vi "WPI_AnalogTriggerVoltsToValue.vi"(8 "error in (no error)":errorcluster, 9 "Voltage":dbl, 10 "AnalogTriggerSource":T1={"Channel"=enum."AI 1", "Averaged"=FALSE, "Filter"=FALSE}, 11 "AnalogTriggerDevRef":T3) -> (0 "error out":errorcluster, 1 "Value":i32, 3 "AnalogTriggerDevRef":T3)   [LabVIEW 2017]
doc: "This software is licensed. Open the labview\\readme\\WPI Robotics Library Open Source License.txt file for more information."
uses:
  <vilib>/Rock Robotics/SystemInterfaces/AnalogTrigger/FPGA_AnalogTriggerDevRef.ctl
  <vilib>/Rock Robotics/SystemInterfaces/AnalogTrigger/FPGA_AnalogTriggerIndex.ctl
  <vilib>/Rock Robotics/SystemInterfaces/AnalogTrigger/FPGA_AnalogTriggerSource.ctl
  <vilib>/Rock Robotics/SystemInterfaces/AI/FPGA_AIChannel.ctl
  <vilib>/Rock Robotics/SystemInterfaces/System/FPGA_SystemGet.vi
  <vilib>/Rock Robotics/SystemInterfaces/AI/FPGA_AIOversampleBits.vi
  <vilib>/Rock Robotics/SystemInterfaces/AI/FPGA_AIERRInvalidAnalogChannel.vi
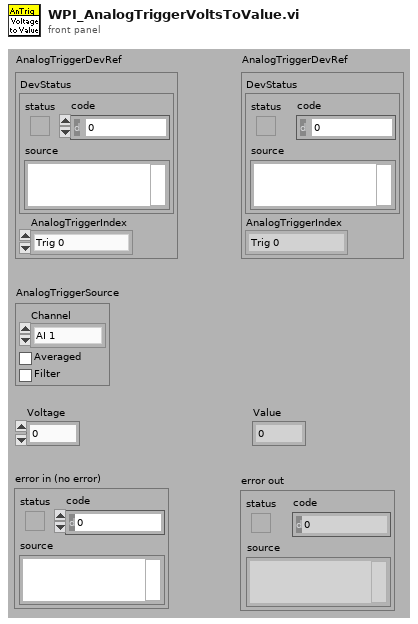
[diagram p1: front panel]
types:
  T1 = typedef "FPGA_AnalogTriggerSource.ctl" = cluster{"Channel":T2, "Averaged":bool, "Filter":bool}
  T2 = typedef "FPGA_AIChannel.ctl" = enum8{"AI 0", "AI 1", "AI 2", "AI 3", "AI MXP 0", "AI MXP 1", "AI MXP 2", "AI MXP 3", "Invalid"}
  T3 = typedef "FPGA_AnalogTriggerDevRef.ctl" = cluster{"DevStatus":errorcluster, "AnalogTriggerIndex":T4}
  T4 = typedef "FPGA_AnalogTriggerIndex.ctl" = enum8{"Trig 0", "Trig 1", "Trig 2", "Trig 3", "Trig 4", "Trig 5", "Trig 6", "Trig 7", "Invalid"}
  T5 = typedef "FPGA_AIDevRef.ctl" = cluster{"DevStatus":errorcluster}
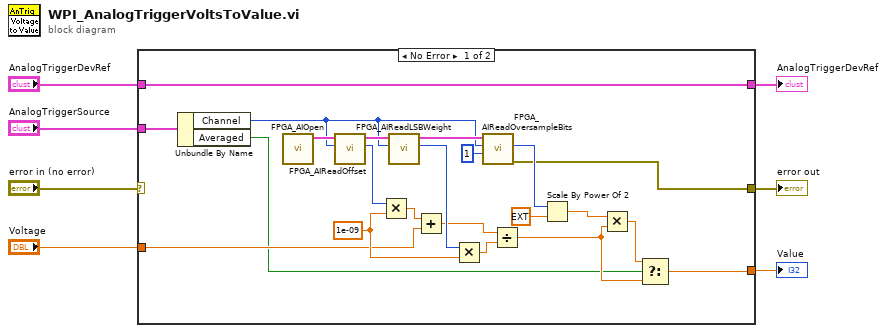
[diagram p0: block diagram]
diagram:
  n1 = case shown="No Error" "error in (no error)" {
    selector: "error in (no error)" -> [_ w30]
    tunnel: "AnalogTriggerDevRef" -> [w12 w31]
    tunnel: [w12 w31] -> w6
    tunnel: [w9 w30] -> w4
    tunnel: "Voltage" -> [w23 _]
    tunnel: [w17 _] -> w2
    tunnel: "AnalogTriggerSource" -> [w11 _]
    frame No Error {
      w29 = 1e-09 ("y")
      n2 = Unbundle By Name(w11) -> ("Channel"=w13:T2, "Averaged"=w10:bool)
      n3 = call <vilib>:"FPGA_AIOpen.vi"() -> ("AI Reference out"=w28:T5)  [unwired: 3 in, 8 out]
      n4 = call <vilib>:"FPGA_AIReadOffset.vi"("Channel"=w13, "AI Reference"=w28) -> ("Offset"=w26:i32, "AI Reference"=w27:T5)  [unwired: 1 in, 7 out]
      n5 = Multiply(x=w26, y=w29) -> (x*y=w24:dbl)
      n6 = call <vilib>:"FPGA_AIReadLSBWeight.vi"("Channel"=w13, "AI Reference"=w27) -> ("LSBWeight"=w25:u32, "AI Reference"=w20:T5)  [unwired: 1 in, 7 out]
      n7 = Add(x=w24, y=w23) -> (x+y=w22:dbl)
      n8 = Multiply(x=w25, y=w29) -> (x*y=w21:dbl)
      n9 = call <vilib>:"FPGA_AIReadOversampleBits.vi"("Additional Depth"=1, "Channel"=w13, "AI Reference in"=w20) -> ("error out"=w9:errorcluster, "OversampleBits"=w15:u8)  [unwired: 1 in, 6 out]
      n10 = Divide(x=w22, y=w21) -> (x/y=w18:dbl)
      n11 = Scale By Power Of 2(n=w15, x=ext 1.0) -> (x*2^n=w16:ext)
      n12 = Multiply(x=w16, y=w18) -> (x*y=w19:ext)
      n13 = Select(t=w19, s=w10, f=w18) -> (s? t:f=w17:ext)
    }
    frame Error {
    }
  }
  "AnalogTriggerDevRef" <- w6
  "error out" <- w4
  "Value" <- w2
